vi "Initialize Simple Explorer.vi"(8 "error in (no error)":errorcluster, 11 "Application Data in":T1={"Item Tree Control"=refnum, "Value Tree Control"=refnum, "DSF Refnum"=refnum, "Top-Level VI"=refnum, "View State"=enum."Tree", "menu reference"=refnum}) -> (0 "error out":errorcluster, 3 "Application Data out":T1={"Item Tree Control"=refnum, "Value Tree Control"=refnum, "DSF Refnum"=refnum, "Top-Level VI"=refnum, "View State"=enum."Tree", "menu reference"=refnum})   [LabVIEW 2019]
uses:
  Development Tools/Data Sharing Configuration Explorer/Source/Main VI/Application Data.ctl
  Development Tools/Data Sharing Configuration Explorer/Source/Main VI/View Mode.ctl
  DSF Core.lvlibp/Classes/Configuration/Configuration Session.lvclass
panel:
  # "App\nData"
  # "App\nData"
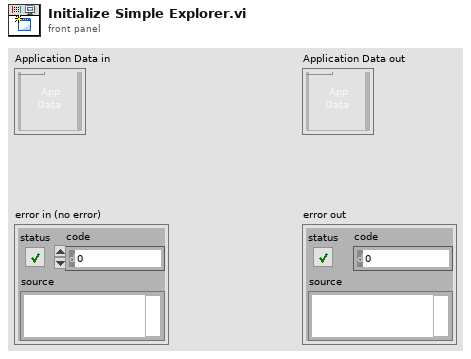
[diagram p1: front panel]
types:
  T1 = typedef "DSF Configuration Utility.lvlib/Application Data.ctl" = cluster{"Item Tree Control":refnum<vi>, "Value Tree Control":refnum<vi>, "DSF Refnum":refnum<class "Configuration Session.lvclass">, "Top-Level VI":refnum<vi>, "View State":T2, "menu reference":refnum<k9>}
  T2 = typedef "DSF Configuration Utility.lvlib/View Mode.ctl" = enum16{"Tree", "List"}
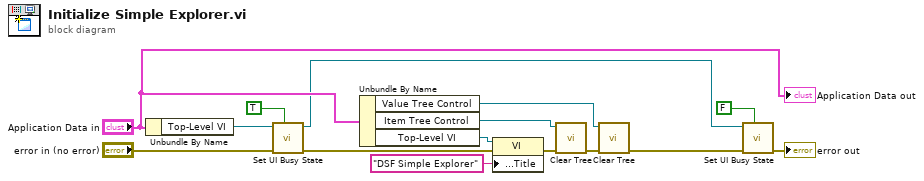
[diagram p0: block diagram]
diagram:
  n1 = Unbundle By Name("Application Data in") -> ("Top-Level VI"=w10:refnum<vi>)
  n2 = call "Set UI Busy State.vi"("Defer Panel Updates"=TRUE, "error in (no error)"="error in (no error)", "VI in"=w10) -> ("error out"=w13:errorcluster, "VI out"=w9:refnum<vi>)  [unwired: 7 in]
  n3 = Unbundle By Name("Application Data in") -> ("Value Tree Control"=w2:refnum<vi>, "Item Tree Control"=w6:refnum<vi>, "Top-Level VI"=w4:refnum<vi>)
  n4 = property class="VI"(reference=w4, error in=w13, "Front Panel.Title"="DSF Simple Explorer" ("Front Panel Window:Title")) -> (error out=w5:errorcluster)  [unwired: 1 out]
  n5 = call "Clear Tree.vi"("error in (no error)"=w5, "TreeControl in"=w6) -> ("error out"=w3:errorcluster)  [unwired: 9 in]
  n6 = call "Clear Tree.vi"("error in (no error)"=w3, "TreeControl in"=w2) -> ("error out"=w14:errorcluster)  [unwired: 9 in]
  n7 = call "Set UI Busy State.vi"("Defer Panel Updates"=FALSE, "error in (no error)"=w14, "VI in"=w9) -> ("error out"=→"error out":errorcluster)  [unwired: 7 in, 1 out]
  "Application Data out" <- "Application Data in"
